vi "CountSurround.vi"(8 "error in":errorcluster, 9 "index Column":i32, 10 "index row":i32, 11 "Array":T1) -> (0 "error out":errorcluster, 1 "Count of 8 Surrounding":i16, 3 "Array Out Unchanged":T1)   [LabVIEW 2018]
uses:
  MainArray.ctl
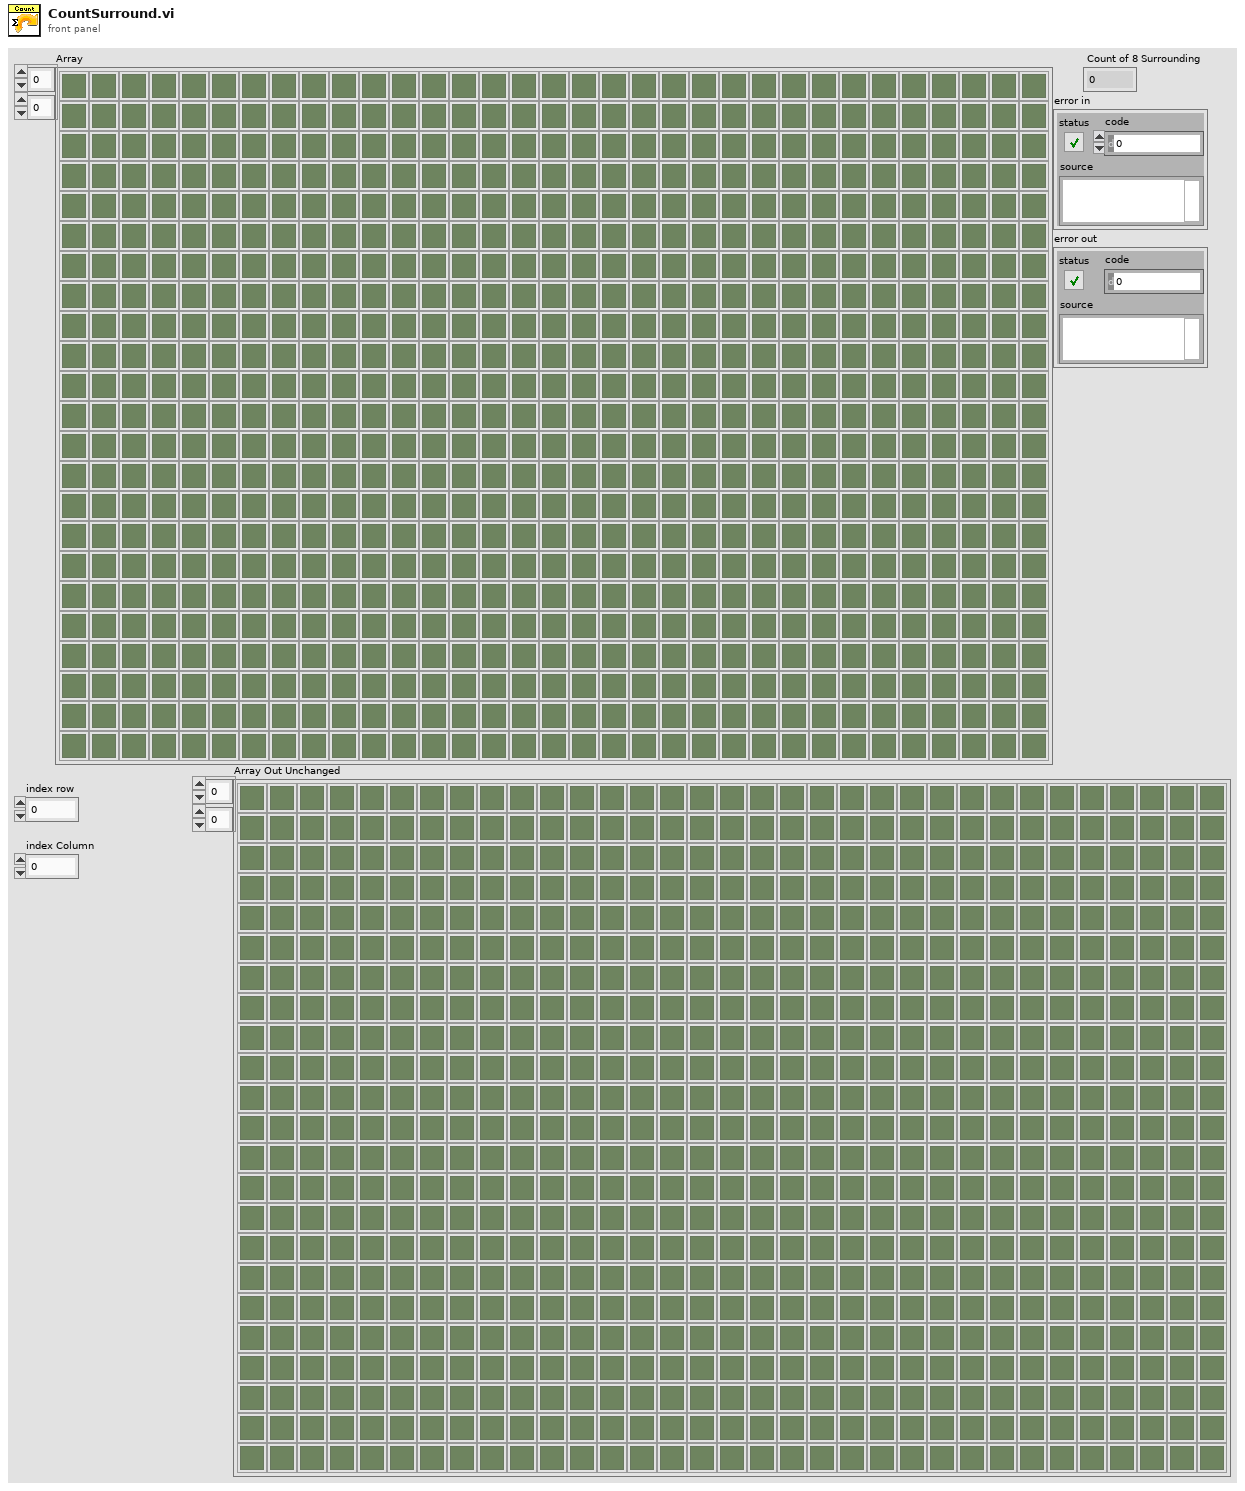
[diagram p1: front panel]
types:
  T1 = typedef "MainArray.ctl" = bool[][]
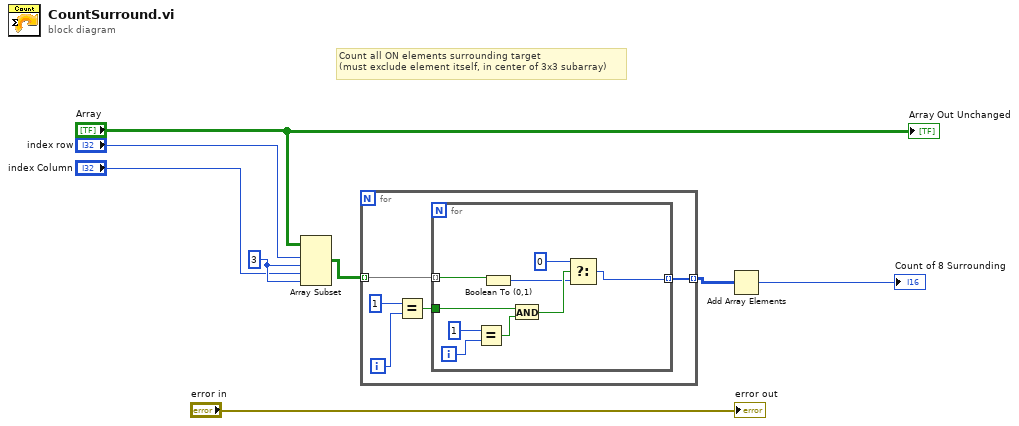
[diagram p0: block diagram]
diagram:
  w8 = 3 ("length")
  # "Count all ON elements surrounding target\n(must exclude element itself, in center of 3x3 subarray)"
  n1 = Array Subset(array="Array", index (row)="index row", length (row)=w8, index (col)="index Column", length (col)=w8) -> (w7:T1)
  n2 = for {
    tunnel: w7 -> [w13] mode=indexing
    tunnel: [w12] -> w4 mode=indexing
    i -> [w11]
    n3 = Equal?(x=1, y=w11) -> (x = y?=w9:bool)
    n4 = for {
      tunnel: w13 -> [w22] mode=indexing
      tunnel: [w16] -> w12 mode=indexing
      tunnel: w9 -> [w18]
      i -> [w20]
      n5 = Equal?(x=1, y=w20) -> (x = y?=w19:bool)
      n6 = Boolean To (0,1)(Boolean=w22) -> (0, 1=w15:i16)
      n7 = And(x=w18, y=w19) -> (x .and. y?=w17:bool)
      n8 = Select(t=i16 0 ("f"), s=w17, f=w15) -> (s? t:f=w16:i16)
    }
  }
  n9 = Add Array Elements(numeric array=w4) -> (sum=→"Count of 8 Surrounding":i16)
  "Array Out Unchanged" <- "Array"
  "error out" <- "error in"
